vi "VI AK TCP - Amium.vi"(6 "Aktionen":T1, 7 "connection ID":refnum<k5>, 8 "error in":errorcluster caption="error out", 9 "Port":u16=3615, 10 "IP-Adresse:":string, 11 "Fehlerzähler":i16) -> (0 "error out":errorcluster, 3 "Fehlerzähler":i16, 4 "Aktionen":T1, 5 "connection ID":refnum<k5>)   [LabVIEW 2020, in "Amium PNS.lvlib" / "AK Kommunikation.lvlib"]
uses:
  AK Kommunikation.lvlib
  Aktionen AK Amium.ctl
  Amium Kommandos verwalten Aktionen.ctl
  TCP Timeout Aktionen - Amium.ctl
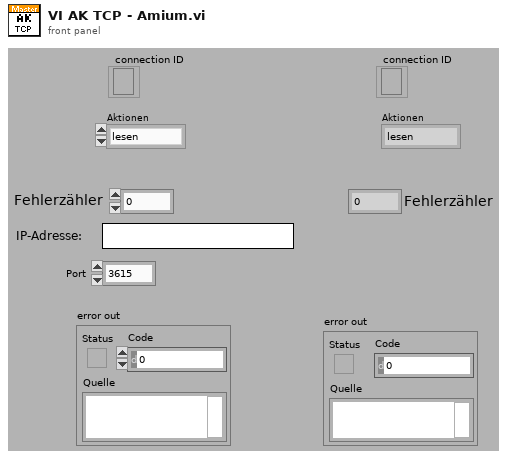
[diagram p1: front panel]
types:
  T1 = typedef "Amium PNS.lvlib/AK Kommunikation.lvlib/Aktionen AK Amium.ctl" = enum16{"lesen", "initialisieren", "beenden", "AK Komm"}
  T2 = typedef "Amium PNS.lvlib/AK Kommunikation.lvlib/TCP Timeout Aktionen - Amium.ctl" = enum16{"lesen", "setzen"}
  T3 = typedef "Amium PNS.lvlib/AK Kommunikation.lvlib/Amium Kommandos verwalten Aktionen.ctl" = enum16{"lesen", "setzen Ende", "setzen Pos1", "senden", "initalisieren", "prüfen", "Kommandos"}
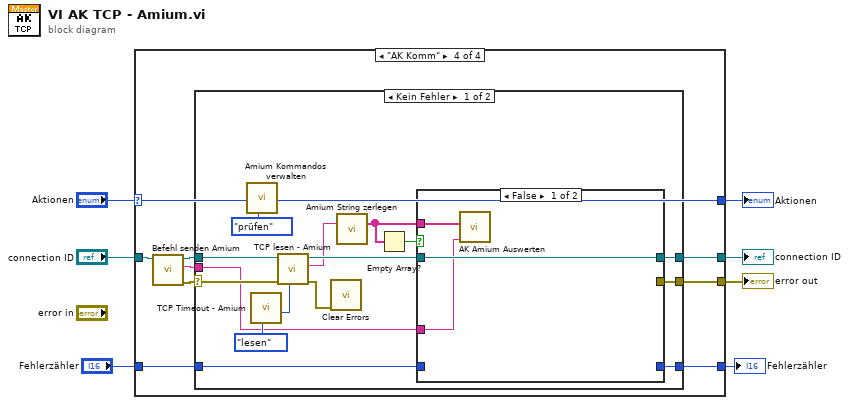
[diagram p0: block diagram]
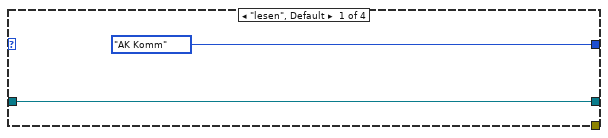
[diagram p2: hidden frame]
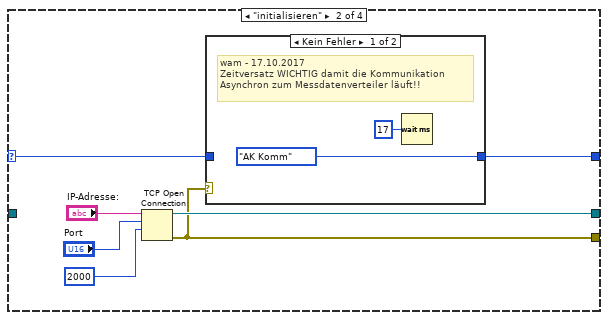
[diagram p3: hidden frame]
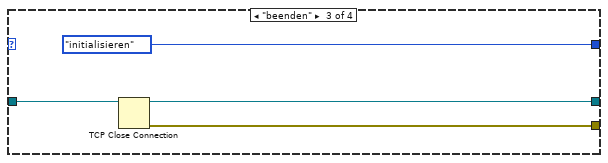
[diagram p5: hidden frame]
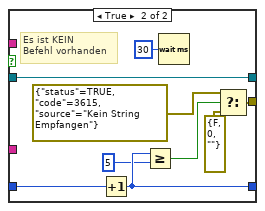
[diagram p6: hidden frame]
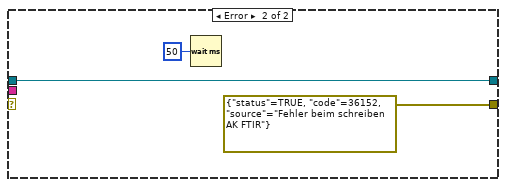
[diagram p7: hidden frame]
diagram:
  n1 = case shown="\"AK Komm\"" "Aktionen" {
    selector: "Aktionen" -> [_ w11 _ w27]
    tunnel: [_ w12 w23 w32] -> w6
    tunnel: [w9 w13 w21 w31] -> w4
    tunnel: "connection ID" -> [w9 _ w22 w30]
    tunnel: [Aktionen_AK_Amium."AK Komm" ("Aktionen") w10 Aktionen_AK_Amium."initialisieren" ("Aktionen") w27] -> w3
    tunnel: [_ _ _ w26] -> w1
    tunnel: "Fehlerzähler" -> [_ _ _ w25]
    frame "lesen", Default {
    }
    frame "initialisieren" {
      n2 = TCP Open Connection(address="IP-Adresse:", remote port or service name="Port", timeout ms (60000)=2000 ("timeout ms (wait forever: -1)")) -> (connection ID=w13:refnum<k5>, error out=w12:errorcluster)  [unwired: 2 in]
      n3 = case shown="Kein Fehler" w12 {
        tunnel: [Aktionen_AK_Amium."AK Komm" ("Aktionen") w19] -> w10
        tunnel: w11 -> [_ w19]
        frame No Error {
          # "wam - 17.10.2017\nZeitversatz WICHTIG damit die Kommunikation \nAsynchron zum Messdatenverteiler läuft!!"
          n4 = Wait (ms)(milliseconds to wait=u32 17 ("Zu wartende ms")) -> ()  [unwired: 1 out]
        }
        frame Error {
        }
      }
    }
    frame "beenden" {
      n5 = TCP Close Connection(connection ID=w22) -> (connection ID out=w21:refnum<k5>, error out=w23:errorcluster)  [unwired: 2 in]
    }
    frame "AK Komm" {
      n6 = call "Befehl senden Amium.vi"("connection ID"=w30) -> ("error out"=w28:errorcluster, "Verknüpfter String"=w24:string, "connection ID"=w29:refnum<k5>)  [unwired: 8 in]
      n7 = case shown="Kein Fehler" w28 {
        selector: w28 -> [w42 _]
        tunnel: [w43 errorcluster {"status"=TRUE, "code"=36152, "source"="Fehler beim schreiben AK FTIR"} ("error out")] -> w32
        tunnel: [w45 w62] -> w31
        tunnel: w29 -> [w44 w62]
        tunnel: [w39 _] -> w26
        tunnel: w25 -> [w38 _]
        tunnel: w24 -> [w33 _]
        frame No Error {
          n8 = call "Amium Kommandos verwalten.vi"("Aktionen"=Amium_Kommandos_verwalten_Aktionen."prüfen") -> ()  [unwired: 8 in, 3 out]
          n9 = call "TCP Timeout - Amium.vi"("Aktionen Timeout"=TCP_Timeout_Aktionen_-_Amium."lesen") -> ("Timeout lesen"=w41:i32)  [unwired: 9 in, 1 out]
          n10 = call "TCP lesen - Amium.vi"("Timeout"=w41, "Fehler (Eingang)"=w42, "connection ID"=w44) -> ("error out"=w40:errorcluster, "Daten (Ausgang)"=w35:string, "connection ID"=w46:refnum<k5>)  [unwired: 6 in]
          n11 = call <vilib>:"Clear Errors.vi"("error in (no error)"=w40) -> ()  [unwired: 5 in, 2 out]
          n12 = call "Amium String zerlegen.vi"("read buffer"=w35) -> ("Array"=w34:string[])  [unwired: 14 in]
          n13 = Empty Array?(array=w34) -> (empty?=w47:bool)
          n14 = case shown="False" w47 {
            tunnel: w34 -> [w49 _]
            tunnel: w46 -> [w50 w59]
            tunnel: [w50 w59] -> w45
            tunnel: [_ w54] -> w43
            tunnel: [_ w56] -> w39
            tunnel: w38 -> [_ w57]
            tunnel: w33 -> [w48 _]
            frame False {
              n15 = call "AK Amium Auswerten.vi"("Verknüpfter String"=w48, "Array"=w49) -> ()  [unwired: 10 in]
            }
            frame True {
              # "Es ist KEIN \nBefehl vorhanden"
              n16 = Increment(x=w57) -> (x+1=w56:i16)
              n17 = Greater Or Equal?(x=w56, y=i16 5) -> (x >= y?=w52:bool)
              n18 = Wait (ms)(milliseconds to wait=u32 30 ("Zu wartende ms")) -> ()  [unwired: 1 out]
              n19 = Select(t=errorcluster {"status"=TRUE, "code"=3615, "source"="Kein String Empfangen"} ("error out"), s=w52, f=errorcluster {"status"=FALSE, "code"=0, "source"=""}) -> (s? t:f=w54:errorcluster)
            }
          }
        }
        frame Error {
          n20 = Wait (ms)(milliseconds to wait=u32 50 ("Zu wartende ms")) -> ()  [unwired: 1 out]
        }
      }
    }
  }
  "error out" <- w6
  "connection ID" <- w4
  "Aktionen" <- w3
  "Fehlerzähler" <- w1
